vi "Configure Channel (TC Scale).vi"(0 "VISA resource name":refnum<visa-resource-name>, 1 "Scaling":T2={"Floating point position (2)"=2, "Lower Scaling (0)"=0.0, "Upper Scaling (100)"=100.0, "Unit Character (\"\")"=""} {"Upper Scaling (100)" format="%_6g"; "Lower Scaling (0)" format="%_6g"; "Floating point position (2)" min=0 max=5 step=1}, 5 "Channel (0001)":string="0001", 7 "Enable Channel (True)":bool=TRUE, 9 "Range and Span":T1={"Thermocouple Type (0 : R)"=0, "Enable Span (False)"=FALSE, "Lower Span (0.0)"=0.0, "Upper Span (1760.0)"=1760.0, "Bias (0)"=0.0} {"Thermocouple Type (0 : R)" items=["R", "S", "B", "K", "K-H", "E", "J", "T", "N", "W", "L", "U", "WRe3-25", "PLATINEL", "PR20-40", "KpvsAu7Fe", "NiNiMo", "WWRe26", "N14", "XK"]; "Bias (0)" min=-999999.0 max=999999.0; "Upper Span (1760.0)" min=-10000.0 max=10000.0 format="%#.1f"; "Lower Span (0.0)" min=-10000.0 max=10000.0 step=0.1 format="%#.1f"}, 11 "error in (no error)":errorcluster) -> (4 "VISA resource name out":refnum<visa-resource-name>, 6 "Channel":string, 15 "error out":errorcluster)   [LabVIEW 2020, in "Yokogawa GX Series.lvlib"]
doc: "Sets the input range as thermocouple.\n\nCommand: SRangeAI"
uses:
  <instrlib>/Yokogawa GX Series/Yokogawa GX Series.lvlib
  <instrlib>/Yokogawa GX Series/Private/TC Range.vi
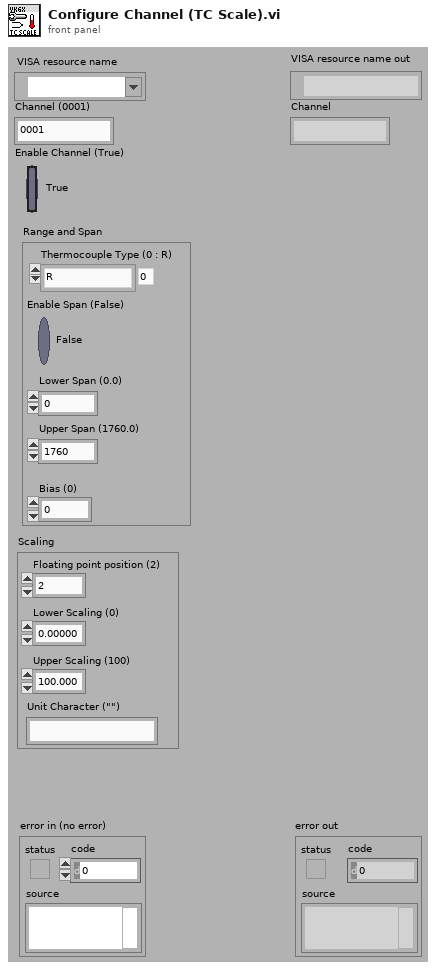
[diagram p1: front panel]
types:
  T1 = cluster{"Thermocouple Type (0 : R)":i32, "Enable Span (False)":bool, "Lower Span (0.0)":dbl, "Upper Span (1760.0)":dbl, "Bias (0)":dbl}
  T2 = cluster{"Floating point position (2)":i32, "Lower Scaling (0)":dbl, "Upper Scaling (100)":dbl, "Unit Character (\"\")":string}
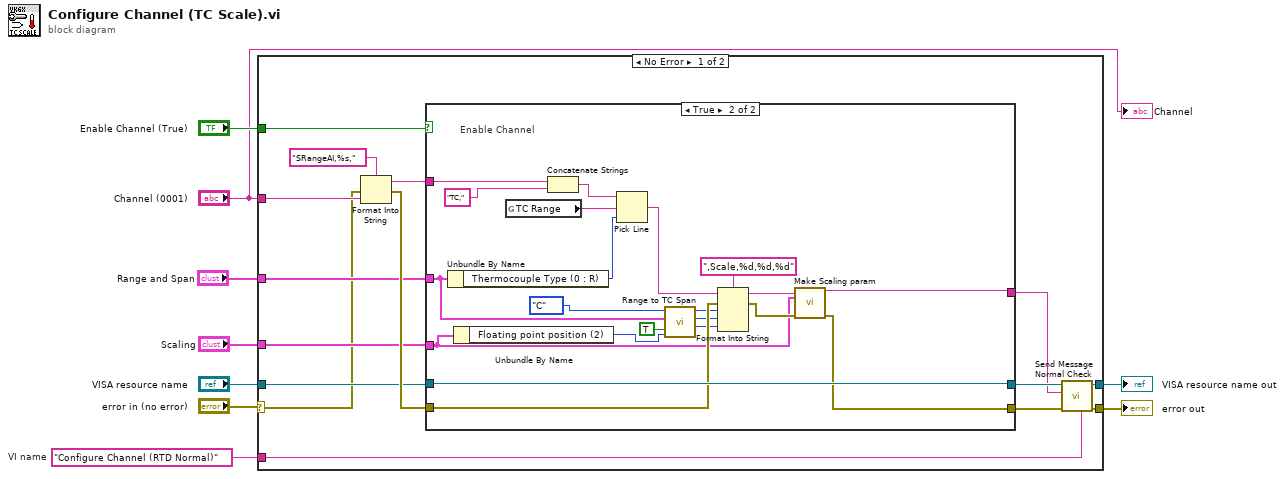
[diagram p0: block diagram]
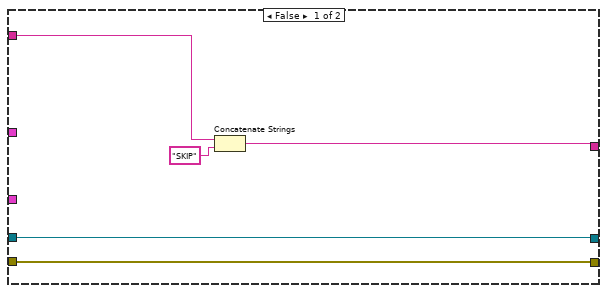
[diagram p2: hidden frame]
diagram:
  w2 = "Configure Channel (RTD Normal)"  # VI name
  n1 = case shown="No Error" "error in (no error)" {
    selector: "error in (no error)" -> [w10 w51]
    tunnel: "Enable Channel (True)" -> [w21 _]
    tunnel: "VISA resource name" -> [w20 w52]
    tunnel: [w16 w52] -> w7
    tunnel: [w15 w51] -> w6
    tunnel: "Scaling" -> [w14 _]
    tunnel: "Range and Span" -> [w13 _]
    tunnel: "Channel (0001)" -> [w12 _]
    tunnel: w2 -> [w11 _]
    frame No Error {
      n2 = Format Into String(format string="SRangeAI,%s,", error in=w10, w12) -> (resulting string=w22:string, error out=w23:errorcluster)  [unwired: 1 in]
      n3 = case shown="True" w21 {
        tunnel: w23 -> [w28 w44]
        tunnel: w22 -> [w29 w49]
        tunnel: [w28 w35] -> w18
        tunnel: w20 -> [w27 w45]
        tunnel: [w27 w45] -> w19
        tunnel: w13 -> [_ w39]
        tunnel: [w25 w36] -> w17
        tunnel: w14 -> [_ w33]
        frame False {
          n4 = Concatenate Strings(w29, "SKIP") -> (w25:string)
        }
        frame True {
          # "Enable Channel"
          n5 = Unbundle By Name(w39) -> ("Thermocouple Type (0 : R)"=w47:i32)
          n6 = Unbundle By Name(w33) -> ("Floating point position (2)"=w32:i32)
          n7 = global read "TC Range.vi" "TC Range"() -> (w30:string)
          n8 = Concatenate Strings(w49, "TC,") -> (w48:string)
          n9 = Pick Line(string ("")=w48, multi-line string=w30, line index=w47) -> (output string=w46:string)
          n10 = call <instrlib>:"Range to TC Span.vi"("Floating Point Position (2)"=w32, "Scaling? (False)"=TRUE, "Range and Span"=w39, "Temp. Unit (0: C)"=enum16{"C", "F"}."C") -> ("Bias"=w40:i32, "Upper Span"=w41:i32, "Lower Span"=w42:i32)  [unwired: 5 in]
          n11 = Format Into String(format string=",Scale,%d,%d,%d", initial string=w46, error in=w44, w42, w41, w40) -> (resulting string=w38:string, error out=w37:errorcluster)
          n12 = call <instrlib>:"Make Scaling param.vi"("String (\"\")"=w38, "Scaling"=w33, "error in (no error)"=w37) -> ("String After"=w36:string, "error out"=w35:errorcluster)  [unwired: 11 in]
        }
      }
      n13 = call <instrlib>:"Send Message Normal Check.vi"("Source (\"\")"=w11, "error in (no error)"=w18, "Send Message (\"\")"=w17, "VISA resource name"=w19) -> ("error out"=w15:errorcluster, "VISA resource name out"=w16:refnum<visa-resource-name>)  [unwired: 2 in, 4 out]
    }
    frame Error {
    }
  }
  "error out" <- w6
  "VISA resource name out" <- w7
  "Channel" <- "Channel (0001)"
